vi "shut off ITC box.vi"(8 "error in":errorcluster, 11 "ITC503 Address":refnum<visa-resource-name>) -> (0 "error out":errorcluster, 3 "ITC503 Address out":refnum<visa-resource-name>)   [LabVIEW 2010]
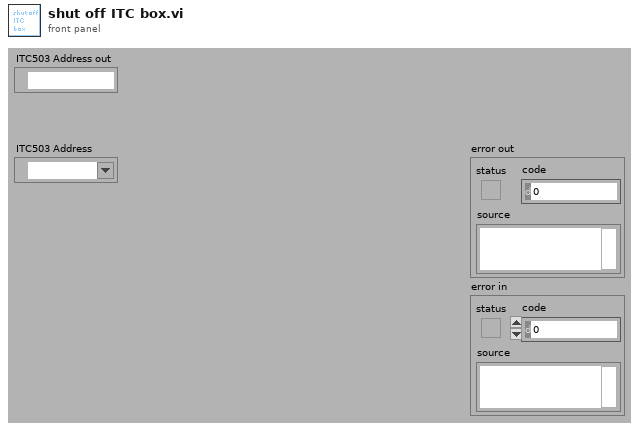
[diagram p1: front panel]
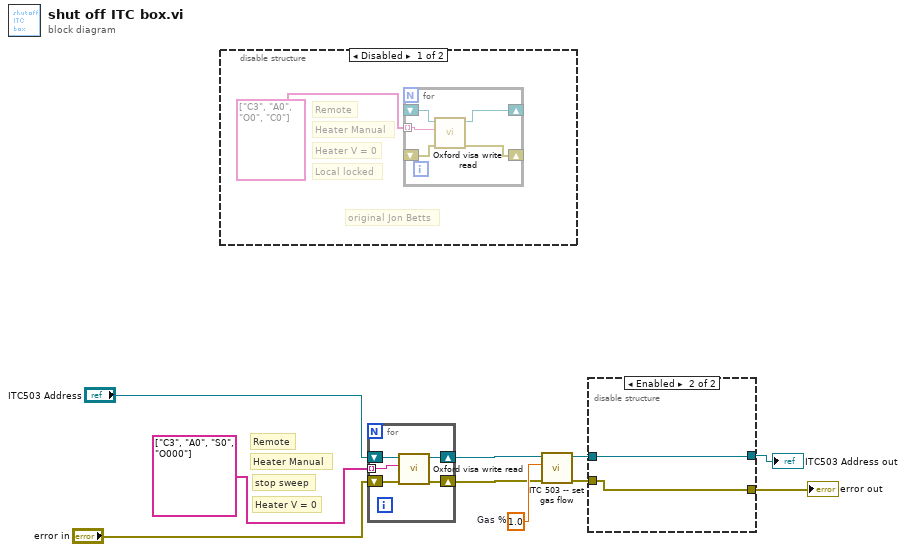
[diagram p0: block diagram]
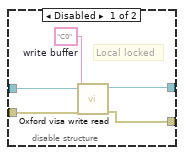
[diagram p2: hidden frame]
diagram:
  w9 = 1.0  # Gas %
  # "stop sweep"
  # "Heater V = 0"
  # "Heater Manual"
  # "Remote"
  n1 = disable-structure shown="Disabled" {
    frame Disabled {
      # "original Jon Betts"
      # "Local locked"
      # "Heater V = 0"
      # "Heater Manual"
      # "Remote"
      n2 = for {
        tunnel: string[] ["C3", "A0", "O0", "C0"] -> [w15] mode=indexing
        shift-right: [w13] -> _
        shift-left: _ -> [w14]
        shift-right: [w12] -> _
        shift-left: _ -> [w16]
        n3 = call "Oxford visa write read.vi"("error in (no error)"=w14, "write buffer"=w15, "VISA resource name"=w16) -> ("error out"=w13:errorcluster, "VISA resource name out"=w12:refnum<visa-resource-name>)  [unwired: 6 in, 1 out]
      }
    }
    frame Enabled {
    }
  }
  n4 = for {
    tunnel: string[] ["C3", "A0", "S0", "O000"] -> [w20] mode=indexing
    shift-right: [w18] -> w8
    shift-left: "ITC503 Address" -> [w21]
    shift-right: [w17] -> w7
    shift-left: "error in" -> [w19]
    n5 = call "Oxford visa write read.vi"("error in (no error)"=w19, "write buffer"=w20, "VISA resource name"=w21) -> ("error out"=w17:errorcluster, "VISA resource name out"=w18:refnum<visa-resource-name>)  [unwired: 6 in, 1 out]
  }
  n6 = call "ITC 503 -- set gas flow.vi"("error in"=w7, "Gas %"=w9, "ITC503 Address"=w8) -> ("error out"=w5:errorcluster, "ITC503 Address OUT"=w6:refnum<visa-resource-name>)  [unwired: 7 in]
  n7 = disable-structure shown="Enabled" {
    disable-tunnel: w6 -> [w25 w28]
    disable-tunnel: w5 -> [w24 w27]
    disable-tunnel: [w23 w28] -> w4
    disable-tunnel: [w22 w27] -> w3
    frame Disabled {
      w26 = "C0"  # write buffer
      # "Local locked"
      n8 = call "Oxford visa write read.vi"("error in (no error)"=w24, "write buffer"=w26, "VISA resource name"=w25) -> ("error out"=w22:errorcluster, "VISA resource name out"=w23:refnum<visa-resource-name>)  [unwired: 6 in, 1 out]
    }
    frame Enabled {
    }
  }
  "error out" <- w3
  "ITC503 Address out" <- w4
